vi "Get Temperature F.vi"(11 "temperature":sgl) -> (2 "function return":u32, 3 "temperature out":sgl)   [LabVIEW 2018, in "Copy of Andor SDK.lvlib"]
doc: "EXPNETTYPE unsigned int WINAPI GetTemperatureF(float * temperature);"
uses:
  Copy of Andor SDK.lvlib
  <userlib>/Andor SDK/ATMCD32D.dll
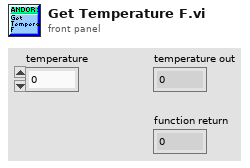
[diagram p1: front panel]
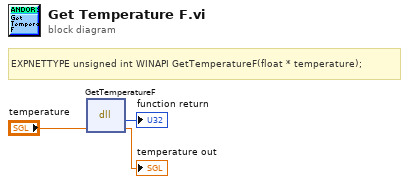
[diagram p0: block diagram]
diagram:
  # "EXPNETTYPE unsigned int WINAPI GetTemperatureF(float * temperature);"
  n1 = dll-call lib="C:/Program Files (x86)/National Instruments/LabVIEW 2018/user.lib/Andor SDK/ATMCD32D.*" fn="GetTemperatureF"("temperature"="temperature") -> (→"function return":u32, "temperature"=→"temperature out":sgl)  [unwired: 3 in, 2 out]
